vi "Create Test Configuration.vi"() -> (0 "error out":errorcluster, 1 "Names":string[](array[string]), 2 "Line Array":T1[](array[typedef]), 3 "Module Configuration":refnum<class "SystemLink configuration.lvclass">, 4 "Channels":refnum<class "TBM channel.lvclass">[](array[class]), 5 "instance identifier":string)   [LabVIEW 2015, in "SystemLink Tag Module tests.lvlib"]
doc: "This VI creates a standard test configuration for other unit tests. It currently creates and adds one line with every datatype to the module configuration."
uses:
  SystemLink Tag Module tests.lvlib
  module/configuration/SystemLink configuration.lvclass
  module/configuration/Line.ctl
  <vilib>/NI/Tag Bus Module Framework/channel/TBM channel.lvclass
  module/configuration/Data Tag Type.ctl
  <vilib>/NI/Tag Bus Module Framework/channel/channel classification.ctl
  module/configuration/Connection Type.ctl
  module/configuration/Connection Configuration.ctl
  module/configuration/SystemLink configuration.lvclass/SystemLink configuration.ctl
  module/configuration/Write Prepend Minion ID.vi
  module/configuration/Write Connection Configuration.vi
  <vilib>/NI/Configuration Framework/serializable configuration/NISE_CEF_serializable configuration.lvclass
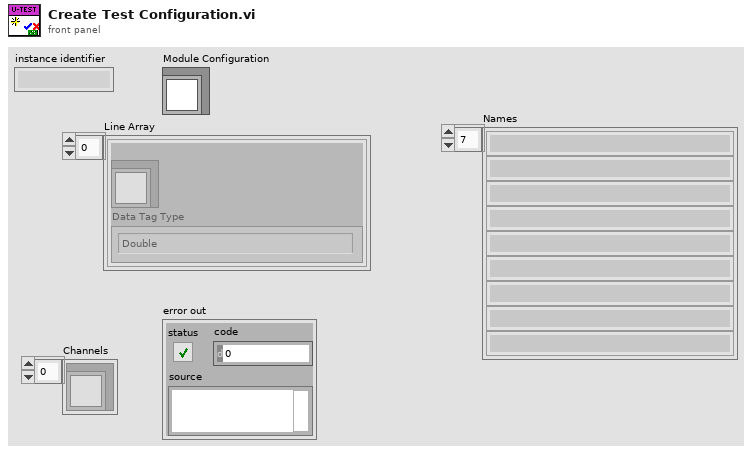
[diagram p1: front panel]
types:
  T1 = typedef "SystemLink configuration.lvclass/Line.ctl" = cluster{"channel":refnum<class "TBM channel.lvclass">, "Data Tag Type":T2}
  T2 = typedef "SystemLink configuration.lvclass/Data Tag Type.ctl" = enum16{"Double", "Single", "I32", "I16", "I8", "U64", "U32", "U16", "U8", "Boolean", "String", "Timestamp"}
  T3 = typedef "SystemLink configuration.lvclass/Connection Configuration.ctl" = cluster{"Connection Type":T4, "AMQP":cluster{"Configuration ID":string}, "HTTP":cluster{"Verify Server?":bool, "Server URL":string, "CA Certificate File":string, "User Info":cluster{"Username":string, "Password":string}, "API Key":string}}
  T4 = typedef "SystemLink configuration.lvclass/Connection Type.ctl" = enum16{"AMQP", "HTTP", "API Key (SystemLink Cloud)"}
  T5 = cluster{"Verify Server?":bool, "Server URL":string, "CA Certificate File":string, "User Info":cluster{"Username":string, "Password":string}, "API Key":string}
  T6 = typedef "TBM channel.lvclass/channel classification.ctl" = enum16{"input data", "output data", "processing parameter", "processing result"}
  T7 = typedef "tag bus.lvlib/tag descriptor.lvclass/Data Type.ctl" = enum16{"Double", "Single", "I64", "I32", "I16", "I8", "U64", "U32", "U16", "U8", "Boolean", "String", "Array of Double", "Array of Single", "Array of I64", "Array of I32", "Array of I16", "Array of I8", "Array of U64", "Array of U32", "Array of U16", "Array of U8", "Array of Boolean", "Array of String"}
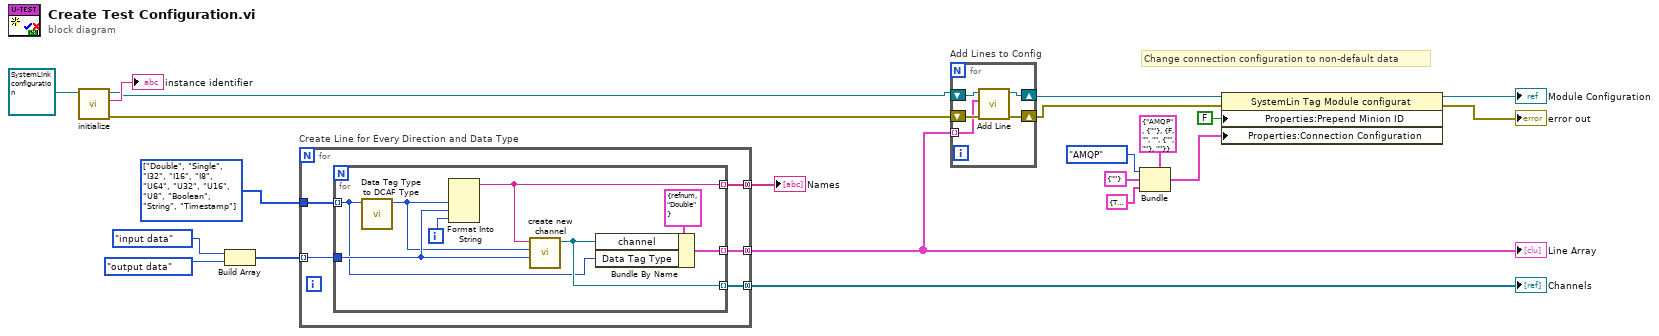
[diagram p0: block diagram]
diagram:
  w12 = T2[] [enum."Double", enum."Single", enum."I32", enum."I16", enum."I8", enum."U64", enum."U32", enum."U16", enum."U8", enum."Boolean", enum."String", enum."Timestamp"] items=["Double", "Single", "I32", "I16", "I8", "U64", "U32", "U16", "U8", "Boolean", "String", "Timestamp"]
  # "Change connection configuration to non-default data"
  n1 = call <vilib>:"initialize.vi"("configuration in"=refnum<class "SystemLink configuration.lvclass"> refnum ("tag bus configurable plugin module configuration")) -> ("error out"=w20:errorcluster, "identifier"=→"instance identifier":string, "configuration out"=w17:refnum<class "SystemLink configuration.lvclass">)  [unwired: 8 in]
  n2 = Build Array(channel_classification."input data" ("channel classification"), channel_classification."output data" ("channel classification")) -> (w16:T6[])
  n3 = for "Create Line for Every Direction and Data Type" {
    tunnel: w16 -> [w26] mode=indexing
    tunnel: [w24] -> w7 mode=concatenating
    tunnel: w12 -> [w25]
    tunnel: [w23] -> w19 mode=concatenating
    tunnel: [w22] -> w13 mode=concatenating
    n4 = for {
      tunnel: w26 -> [w32]
      tunnel: [w34] -> w24 mode=indexing
      tunnel: w25 -> [w29] mode=indexing
      tunnel: [w31] -> w23 mode=indexing
      tunnel: [w33] -> w22 mode=indexing
      i -> [w27]
      n5 = call "Data Tag Type to DCAF Type.vi"("Data Tag Type"=w29) -> ("DCAF Data Type"=w30:T7)  [unwired: 10 in]
      n6 = Format Into String(w30, w32, w27) -> (resulting string=w31:string)  [unwired: 3 in, 1 out]
      n7 = call <vilib>:"create new channel.vi"("channel classification"=w32, "data type"=w30, "channel name"=w31) -> ("channel"=w33:refnum<class "TBM channel.lvclass">)  [unwired: 8 in]
      n8 = Bundle By Name(cluster=T1 {"channel"=refnum, "Data Tag Type"=enum."Double"} ("Line"), "channel"=w33, "Data Tag Type"=w29) -> (w34:T1)
    }
  }
  "Names" <- w19
  "Line Array" <- w7
  "Channels" <- w13
  n9 = for "Add Lines to Config" {
    tunnel: w7 -> [w35] mode=indexing
    shift-right: [w38] -> w9
    shift-left: w17 -> [w39]
    shift-right: [w36] -> w8
    shift-left: w20 -> [w37]
    n10 = call "Add Line.vi"("error in"=w37, "Line"=w35, "SystemLin Tag Module configuration in"=w39) -> ("error out"=w36:errorcluster, "SystemLin Tag Module configuration out"=w38:refnum<class "SystemLink configuration.lvclass">)  [unwired: 6 in, 1 out]
  }
  n11 = Bundle(cluster=T3 {"Connection Type"=enum."AMQP", "AMQP"={"Configuration ID"=""}, "HTTP"={"Verify Server?"=FALSE, "Server URL"="", "CA Certificate File"="", "User Info"={"Username"="", "Password"=""}, "API Key"=""}} ("Connection Configuration"), "Connection Type"=Connection_Type."AMQP", "AMQP"=cluster{"Configuration ID":string} {"Configuration ID"=""}, "HTTP"=T5 {"Verify Server?"=TRUE, "Server URL"="Server URL", "CA Certificate File"="\\ni-rt\\system", "User Info"={"Username"="username", "Password"="password"}, "API Key"="API Key"}) -> (w2:T3)
  n12 = property class="SystemLin Tag Module configurat"(reference=w9, error in=w8, "Properties:Prepend Minion ID"=FALSE ("Prepend Minion ID"), "Properties:Connection Configuration"=w2) -> (reference out=→"Module Configuration":refnum<class "SystemLink configuration.lvclass">, error out=→"error out":errorcluster)
